vi "CH_LM get Meter Info.vi"(8 "error in (no error)":errorcluster, 11 "Meter Index":i32) -> (0 "error out":errorcluster, 1 "Meter Info":T1, 2 "Serial Number out":string, 3 "Meter Index out":i32, 4 "All Meter Infos":T1[](array[typedef]), 5 "All Meter Indices":i32[](array[numeric]), 6 "All Serial Numbers":string[](array[string]))   [LabVIEW 2017, in "CH_LM.lvlib"]
doc: "This VI reads meter infos from private FGV."
uses:
  CH_LM.lvlib
  CH_LM Meter Info.ctl
  _CH_LM/CH_LM Queue Cluster.ctl
  _CH_LM/CH_LM Event Cluster.ctl
  CH_LM Data Token.ctl
  _CH_LM/CH_LM Action Enumeration.ctl
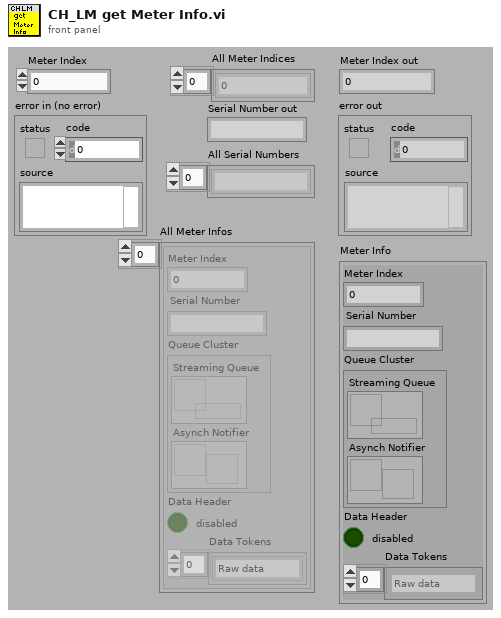
[diagram p1: front panel]
types:
  T1 = typedef "CH_LM.lvlib/CH_LM Meter Info.ctl" = cluster{"Meter Index":i32, "Serial Number":string, "Queue Cluster":T2, "Data Header":bool, "Data Tokens":T3[]}
  T2 = typedef "CH_LM.lvlib/CH_LM Queue Cluster.ctl" = cluster{"Streaming Queue":refnum<queue>, "Asynch Notifier":refnum<notifier>}
  T3 = typedef "CH_LM.lvlib/CH_LM Data Token.ctl" = enum16{"Raw data", "Quad distance", "Formated data", "Unit", "Pulse period", "Flags", "Sequence ID"}
  T4 = typedef "CH_LM.lvlib/CH_LM Action Enumeration.ctl" = enum16{"add", "read", "read by serial", "set", "remove", "delete", "Clear Shift-Register", ""}
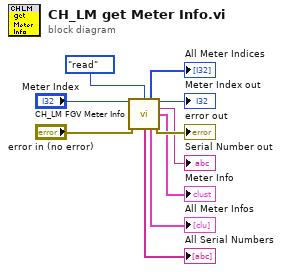
[diagram p0: block diagram]
diagram:
  n1 = call "CH_LM FGV Meter Info.vi"("Meter Index"="Meter Index", "Action (read)"=CH_LM_Action_Enumeration."read", "error in (no error)"="error in (no error)") -> ("All Meter Indices"=→"All Meter Indices":i32[], "Meter Index out"=→"Meter Index out":i32, "Serial Number out"=→"Serial Number out":string, "Meter Info"=→"Meter Info":T1, "All Serial Numbers"=→"All Serial Numbers":string[], "All Meter Infos"=→"All Meter Infos":T1[], "error out"=→"error out":errorcluster)  [unwired: 2 in, 4 out]
